vi "Set_Table_RowCell_Value.vi"(0 "测试信息 2":refnum<vi>, 1 "索引 (行)":i32, 2 "禁用的索引 (列)":i32, 3 "新元素/子数组":string, 5 "error in (no error)":errorcluster caption="错误输入（无错误）") -> (14 "引用输出":refnum<vi>, 19 "error out":errorcluster caption="错误输出")   [LabVIEW 2018]
panel:
  in  "测试信息":i32(listbox)
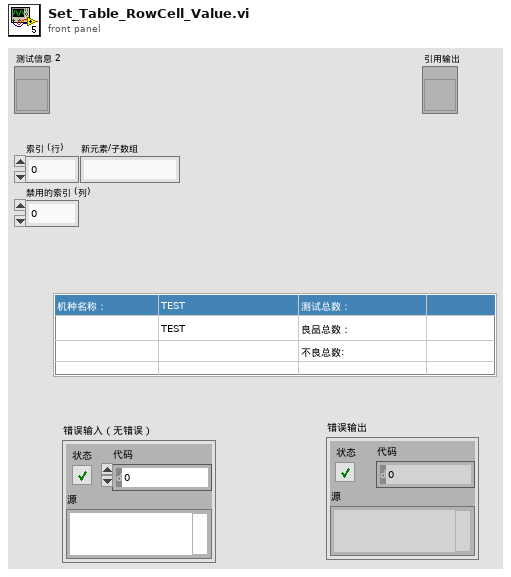
[diagram p1: front panel]
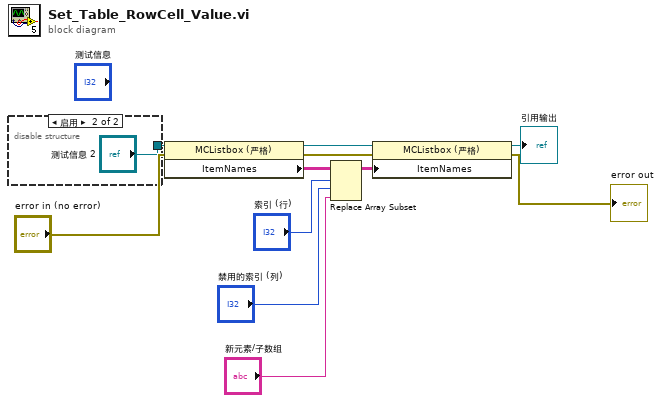
[diagram p0: block diagram]
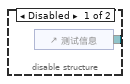
[diagram p2: hidden frame]
diagram:
  n1 = disable-structure shown="启用" {
    disable-tunnel: [w12 "测试信息 2"] -> w11
    frame Disabled {
      n2 = control-ref of="测试信息"() -> (w12:refnum<vi>)
    }
    frame Enabled {
    }
  }
  n3 = property class="MCListbox (严格)"(reference=w11, error in="error in (no error)") -> (reference out=w9:refnum<vi>, error out=w1:errorcluster, "ItemNames"=w10:string[][])
  n4 = Replace Array Subset(array=w10, new element="新元素/子数组", index (row)="索引 (行)", index (col)="禁用的索引 (列)") -> (w8:string[][])
  n5 = property class="MCListbox (严格)"(reference=w9, error in=w1, "ItemNames"=w8) -> (reference out=→"引用输出":refnum<vi>, error out=→"error out":errorcluster)
